vi "Binary to Images V2.vi"() -> ()   [LabVIEW 2013]
panel:
  out "Image/Sector Size(bytes)":i64
  in  "stop":bool
  out "Progress":u64(slide) max=5098 scale=0.0..763.0
  out "Partial images in file?":bool
  out "# of Images":u32
  out "error IO":errorcluster
  out "Height":u32
  out "Width":u32
  in  "Created Image Path":path
  in  "Binary File":path
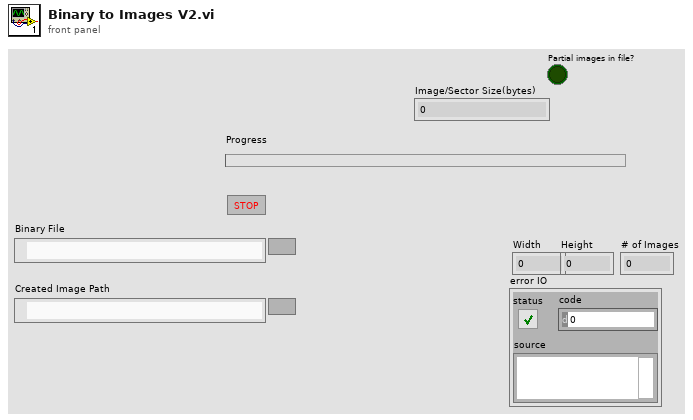
[diagram p1: front panel]
types:
  T1 = typedef "Image Type" = u32
  T2 = typedef "Mask ROI Cluster.ctl" = cluster{"left annulus":T3, "right annulus":T3, "Threshold Range":cluster{"Lower value":dbl, "Upper value":dbl}, "[Avg BG]":u8[], "Number of Sectors":u8, "Left ROI":T4, "Right ROI":T4, "Left Start Angle Duty Cycle":fxp<+,8,0>, "Left End Angle Duty Cycle":fxp<+,8,0>, "Right End Angle Duty Cycle":fxp<+,8,0>, "Right Start Angle Duty Cycle":fxp<+,8,0>, "[Sector ROIs]":T4[], "Consecutive Sector Threshold":u8}
  T3 = typedef "IMAQ Circle" = cluster{"Center X":i32, "Center Y":i32, "Inner Radius":i32, "Outer Radius":i32, "Start Angle":dbl, "End Angle":dbl}
  T4 = typedef "ROI Descriptor" = cluster{"Global Rectangle":i32[], "Contours":cluster{"ID":enum32{"External", "Internal"}, "Type":u32, "Coordinates":i32[]}[]}
  T5 = typedef "IMAQ Image.ctl" = refnum<image>
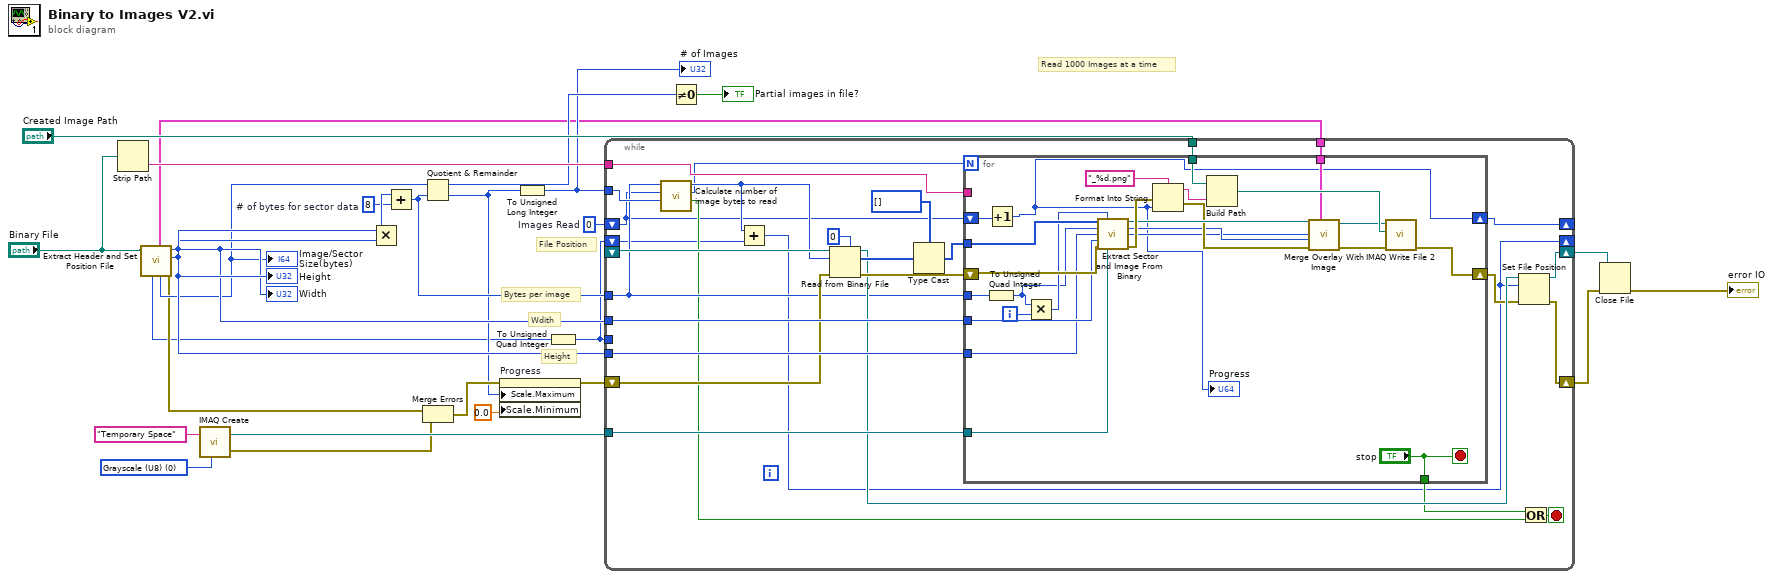
[diagram p0: block diagram]
diagram:
  w6 = u32 0  # Images Read
  w12 = u32 8  # # of bytes for sector data
  w27 = T1 0 items=["Grayscale (U8)", "Grayscale (I16)", "Grayscale (SGL)", "Complex (CSG)", "RGB (U32)", "HSL (U32)", "RGB (U64)", "Grayscale (U16)"] ("Image Type")
  # "Height"
  # "Wdith"
  # "Bytes per image"
  # "File Position"
  # "Read 1000 Images at a time"
  n1 = Strip Path(path="Binary File") -> (name=w23:string)  [unwired: 1 out]
  n2 = call "Extract Header and Set Position File.vi"("Binary File"="Binary File") -> ("error out"=w7:errorcluster, "Height"=w10:u32, "Width"=w9:u32, "Image/Sector Size(bytes)"=w8:i64, "Mask ROI Out"=w1:T2, "Header Size"=w3:i32)  [unwired: 4 in, 1 out]
  "Width" <- w9
  "Height" <- w10
  "Image/Sector Size(bytes)" <- w8
  n3 = call "IMAQ Create"("Image Name"="Temporary Space", "Image Type"=w27) -> ("New Image"=w26:T5, "error out"=w25:errorcluster)  [unwired: 3 in]
  n4 = Multiply(x=w10, y=w9) -> (x*y=w13:u32)
  n5 = Add(x=w13, y=w12) -> (x+y=w11:u32)
  n6 = Quotient & Remainder(x=w8, y=w11) -> (x-y*floor(x/y)=w19:i64, floor(x/y)=w5:i64)
  n7 = Merge Errors(w7, w25) -> (w17:errorcluster)
  n8 = property on="Progress" class="Slide (strict)"(error in=w17, "Scale.Maximum"=w5, "Scale.Minimum"=0.0 ("Data Entry Limits:Minimum")) -> (error out=w16:errorcluster)  [unwired: 1 in, 1 out]
  n9 = To Unsigned Long Integer(number=w5) -> (unsigned 32bit integer=w4:u32)
  "# of Images" <- w4
  n10 = To Unsigned Quad Integer(1:w3) -> (0:w2:u64)
  n11 = while {
    tunnel: w26 -> [w56]
    tunnel: "Created Image Path" -> [w55]
    tunnel: w23 -> [w54]
    tunnel: w9 -> [w53]
    tunnel: w10 -> [w52]
    shift-right: [w45] -> w21
    shift-left: w16 -> [w50]
    shift-right: [w43] -> w18
    shift-left: _ -> [w51]
    tunnel: w11 -> [w41]
    tunnel: w2 -> [_]
    shift-right: [w33] -> _
    shift-left: w6 -> [w34]
    tunnel: w4 -> [w42]
    shift-right: [w30] -> _
    shift-left: w2 -> [w38]
    tunnel: w1 -> [w29]
    stop <- w39 stop-if-true
    n12 = call "Calculate number of image bytes to read.vi"("# of total images"=w42, "Total Images Read"=w34, "# of bytes per image"=w41) -> ("All Images Read?"=w40:bool, "# of Images Read"=w35:u32, "# of bytes to read"=w37:u64)  [unwired: 6 in]
    n13 = Add(x=w37, y=w38) -> (x+y=w30:u64)
    n14 = Read from Binary File(5:u8 0, 8:w50, 10:w37, 11:w51) -> (0:w49:errorcluster, 2:w47:u8[], 3:w44:refnum<file>)  [unwired: 2 in, 1 out]
    n15 = Type Cast(type=u64[] [], x=w47) -> (*(type *) &x=w36:u64[])
    n16 = for {
      N: w35 -> [_]
      tunnel: w56 -> [w68]
      tunnel: w55 -> [w81]
      tunnel: w54 -> [_]
      tunnel: w53 -> [w70]
      tunnel: w52 -> [w69]
      tunnel: w41 -> [w76]
      tunnel: w36 -> [w73]
      shift-right: [w57] -> w33
      shift-left: w34 -> [w66]
      shift-right: [w77] -> w32
      shift-left: w49 -> [w74]
      tunnel: ["stop"] -> w31
      tunnel: w29 -> [w60]
      i -> [w75]
      stop <- "stop" stop-if-true
      n17 = To Unsigned Quad Integer(1:w76) -> (0:w71:u64)
      n18 = Increment(x=w66) -> (x+1=w57:u32)
      "Progress" <- w57
      n19 = Multiply(x=w71, y=w75) -> (x*y=w72:u64)
      n20 = call "Extract Sector and Image From Binary.vi"("Binary Data"=w73, "Start Index"=w72, "# of bytes per image"=w71, "Height"=w69, "Width"=w70, "error in (no error)"=w74, "Image Destination"=w68) -> ("Image Out"=w64:T5, "Left Sector"=w59:u16, "Right Sector"=w58:u16, "error out"=w67:errorcluster)  [unwired: 5 in]
      n21 = Format Into String(format string="_%d.png", error in=w67, w57) -> (resulting string=w79:string, error out=w61:errorcluster)  [unwired: 1 in]
      n22 = Build Path(base path=w81, name or relative path=w79) -> (appended path=w78:path)
      n23 = call "Merge Overlay With Image.vi"("ROI Cluster"=w60, "Error in"=w61, "Left Edge"=w59, "Right Edge"=w58, "Image In"=w64) -> ("error out"=w62:errorcluster, "Image Out"=w63:T5)  [unwired: 5 in]
      n24 = call-poly "IMAQ Write File 2"("error in (no error)"=w62, "File Path"=w78, "Image"=w63) -> ("error out"=w77:errorcluster)  [unwired: 7 in, 1 out]
    }
    n25 = Set File Position(offset (in bytes) (0)=w30, refnum=w44, error in=w32) -> (refnum out=w43:refnum<file>, error out=w45:errorcluster)  [unwired: 1 in]
    n26 = Or(x=w31, y=w40) -> (x .or. y?=w39:bool)
  }
  n27 = Not Equal To 0?(x=w19) -> (x != 0?=→"Partial images in file?":bool)
  n28 = Close File(refnum=w18, error in=w21) -> (error out=→"error IO":errorcluster)  [unwired: 1 out]
